vi "Day of year to Timestamp.vi"(4 "Year (1904-2040)":i32=1904 min=1904 max=2040 step=1, 5 "Julian Day (1-366)":i32=1 min=1 max=366 step=1) -> (2 "Georgian Date":string)   [LabVIEW 2011]
doc: "Converts Julian Date to Georgian Date String."
panel:
  out "time stamp":timestamp
  in  "date time rec":T1={"second"=0, "minute"=0, "hour"=0, "day of month"=60, "month"=0, "year"=2004, "day of week"=0, "day of year"=0, "is DST"=0}
  # "Julian to Georgian Date Conversion"
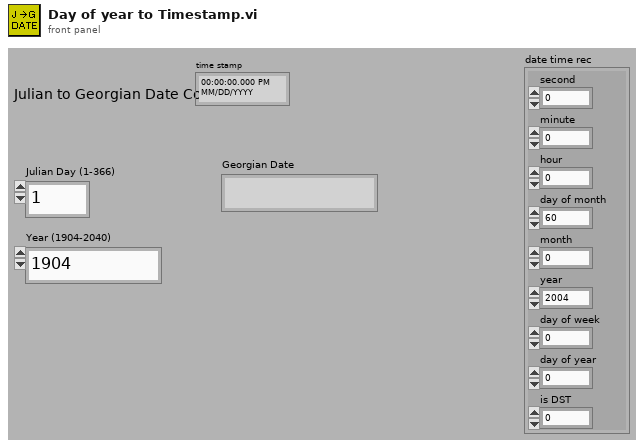
[diagram p1: front panel]
types:
  T1 = cluster{"second":i32, "minute":i32, "hour":i32, "day of month":i32, "month":i32, "year":i32, "day of week":i32, "day of year":i32, "is DST":i32}
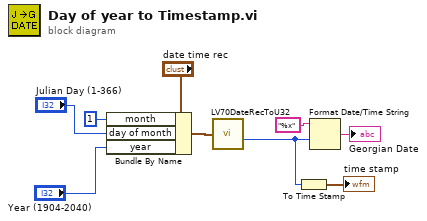
[diagram p0: block diagram]
diagram:
  n1 = Bundle By Name(cluster="date time rec", "month"=1, "day of month"="Julian Day (1-366)", "year"="Year (1904-2040)") -> (w3:T1)
  n2 = call <vilib>:"LV70DateRecToU32.vi"("date time rec"=w3) -> ("Time"=w2:u32)
  n3 = To Time Stamp(1:w2) -> (0:→"time stamp":timestamp)
  n4 = Format Date/Time String(time format string (%c)="%x", seconds (now)=w2) -> (date/time string=→"Georgian Date":string)  [unwired: 1 in]
